vi "Actor Core.vi"(8 "error in":errorcluster, 11 "DisplayWindow in":refnum<class "DisplayWindow.lvclass">) -> (0 "error out":errorcluster, 3 "Actor out":refnum<class "Actor.lvclass">)   [LabVIEW 2016, in "DisplayWindow.lvlib" / "DisplayWindow.lvclass"]
doc: "(<B>Filename</B>: Actor Framework.lvlib:Actor.lvclass:Actor Core.vi)\n\nReceives messages to the actor, reacts to them, and initiates any error handling that may shut the actor down.\n\nDescendant classes may override this VI to append parallel tasks for the actor to complete while it handles messages. Overrides use the Call Parent Method node."
uses:
  DisplayWindow.lvclass
  C:/Program Files (x86)/National Instruments/LabVIEW 2016/vi.lib/ActorFramework/Actor/Actor.lvclass
  <vilib>/ActorFramework/Actor/Actor.lvclass
  CrossIcon.ctl
  CheckIcon.ctl
  MoveIcon.ctl
  DisplayWindow.lvclass/DisplayWindow.ctl
  <vilib>/ActorFramework/Actor/Actor.lvclass/Actor.ctl
  <vilib>/ActorFramework/Message Enqueuer/Message Enqueuer.lvclass/Message Enqueuer.ctl
  <vilib>/ActorFramework/Message Enqueuer/Init from Existing Queue.vi
  <vilib>/ActorFramework/Message Enqueuer/Enqueue.vi
  <vilib>/ActorFramework/Stop Msg/Stop Msg.lvclass
  C:/Program Files (x86)/National Instruments/LabVIEW 2016/vi.lib/ActorFramework/Message/Message.lvclass
  <vilib>/ActorFramework/Message Priority Queue/Priority Enqueue.vi
  <vilib>/ActorFramework/Message Enqueuer/Message Enqueuer.lvclass
panel:
  in  "Listbox":i32(listbox)
  in  "move":T1
  in  "chk":T2
  in  "exit":T3
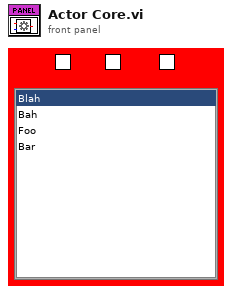
[diagram p1: front panel]
types:
  T1 = typedef "MoveIcon.ctl" = bool
  T2 = typedef "CheckIcon.ctl" = bool
  T3 = typedef "CrossIcon.ctl" = bool
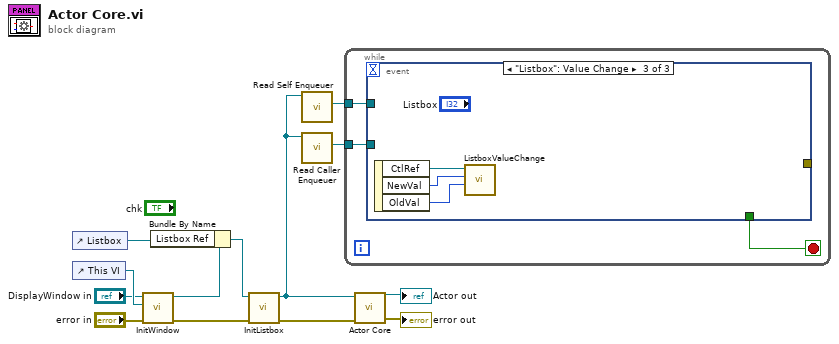
[diagram p0: block diagram]
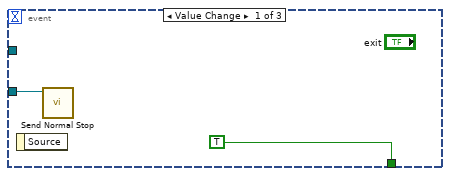
[diagram p2: hidden frame]
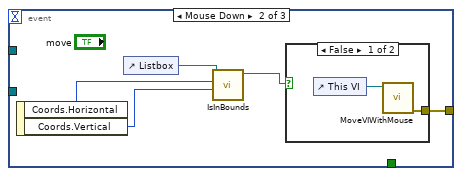
[diagram p3: hidden frame]
diagram:
  n1 = control-ref of="Listbox"() -> (w4:refnum<vi>)
  n2 = control-ref of="This VI"() -> (w11:refnum<vi>)
  n3 = call "InitWindow.vi"("error in (no error)"="error in", "This VI"=w11, "DisplayWindow in"="DisplayWindow in") -> ("error out"=w8:errorcluster, "DisplayWindow out"=w6:refnum<class "DisplayWindow.lvclass">)  [unwired: 7 in]
  n4 = Bundle By Name(cluster=w6, "Listbox Ref"=w4) -> (w2:refnum<class "DisplayWindow.lvclass">)
  n5 = call "InitListbox.vi"("error in (no error)"=w8, "DisplayWindow in"=w2) -> ("error out"=w3:errorcluster, "DisplayWindow out"=w1:refnum<class "DisplayWindow.lvclass">)  [unwired: 8 in]
  n6 = call <vilib>:"Read Self Enqueuer.vi"("Actor"=w1) -> ("Self Enqueuer"=w7:refnum<class "Message Enqueuer.lvclass">)  [unwired: 10 in]
  n7 = call <vilib>:"Read Caller Enqueuer.vi"("Actor"=w1) -> ("Caller Enqueuer"=w5:refnum<class "Message Enqueuer.lvclass">)  [unwired: 10 in]
  n8 = while {
    tunnel: w7 -> [w16]
    tunnel: w5 -> [w15]
    stop <- w14 stop-if-true
    n9 = event shown="[2] \"Listbox\": Value Change" {
      selector: _ -> [_ _ _]
      dyn-events: _ -> [_ _ _]
      timeout: _ -> [_ _ _]
      tunnel: w16 -> [_ _ _]
      tunnel: w15 -> [w18 _ _]
      tunnel: [TRUE _ _] -> w14
      tunnel: [_ w23 _] -> _
      event Value Change {
        n10 = event-data() -> ()  [unwired: 1 in, 1 out]
        n11 = call <vilib>:"Send Normal Stop.vi"("Message Enqueuer"=w18) -> ()  [unwired: 10 in, 1 out]
      }
      event Mouse Down {
        n12 = event-data() -> ("Coords.Horizontal"=w20:i32, "Coords.Vertical"=w21:i32)  [unwired: 1 in]
        n13 = control-ref of="Listbox"() -> (w19:refnum<vi>)
        n14 = call "IsInBounds.vi"("Vertical"=w21, "Horizontal"=w20, "ListBox in"=w19) -> ("Boolean"=w22:bool)  [unwired: 8 in]
        n15 = case shown="False" w22 {
          tunnel: [w24 _] -> w23
          frame False {
            n16 = control-ref of="This VI"() -> (w25:refnum<vi>)
            n17 = call "MoveVIWithMouse.vi"("VI Ref"=w25) -> ("error out"=w24:errorcluster)  [unwired: 10 in]
          }
          frame True {
          }
        }
      }
      event "Listbox": Value Change {
        n18 = event-data() -> ("CtlRef"=w26:refnum<vi>, "NewVal"=w28:i32, "OldVal"=w27:i32)  [unwired: 1 in]
        n19 = call "ListboxValueChange.vi"("OldVal"=w27, "NewVal"=w28, "ListBox in"=w26) -> ()  [unwired: 8 in, 1 out]
      }
    }
  }
  n20 = call-parent "Actor Core.vi"("error in"=w3, "Actor in"=w1) -> ("error out"=→"error out":errorcluster, "Actor out"=→"Actor out":refnum<class "Actor.lvclass">)  [unwired: 8 in]
